vi "SCD - Generate FITS Timestamped File Paths.vi"(8 "error in":errorcluster, 11 "Base Path":path=path "G:/SCD Data/Level-0") -> (0 "error out":errorcluster, 3 "FITS File Path":path=path "G:/SCD Data/Level-0/20141031/20141031T094817.fits")   [LabVIEW 2014]
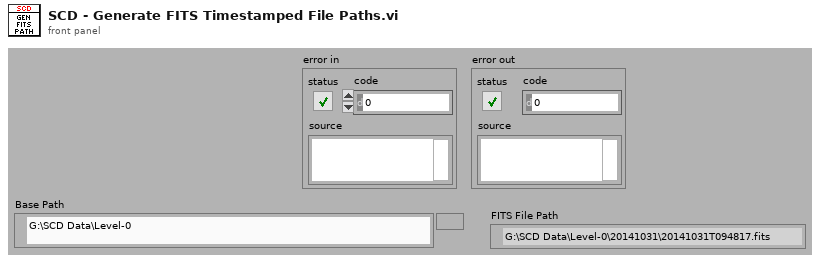
[diagram p1: front panel]
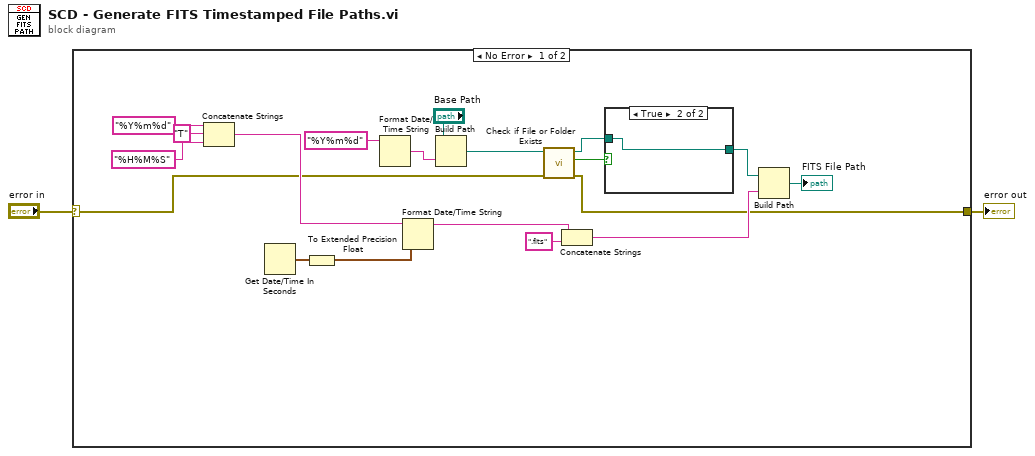
[diagram p0: block diagram]
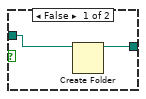
[diagram p2: hidden frame]
diagram:
  n1 = case shown="No Error" "error in" {
    selector: "error in" -> [w4 w24]
    tunnel: [w3 w24] -> w2
    frame No Error {
      n2 = Concatenate Strings("%Y%m%d" ("time format string (%c)"), "T" ("time format string (%c)"), "%H%M%S" ("time format string (%c)")) -> (w6:string)
      n3 = Get Date/Time In Seconds() -> (seconds since 1Jan1904=w10:timestamp)
      n4 = To Extended Precision Float(1:w10) -> ()  [unwired: 1 out]
      n5 = Format Date/Time String(time format string (%c)="%Y%m%d") -> (date/time string=w16:string)  [unwired: 2 out]
      n6 = Format Date/Time String(time format string (%c)=w6, seconds (now)=w10) -> (date/time string=w12:string)  [unwired: 1 in]
      n7 = Build Path(base path="Base Path", name or relative path=w16) -> (appended path=w19:path)
      n8 = call <vilib>:"Check if File or Folder Exists.vi"("error in (no error)"=w4, "path"=w19) -> ("error out"=w3:errorcluster, "file or folder exists?"=w13:bool, "dup path"=w18:path)  [unwired: 7 out]
      n9 = Concatenate Strings(w12, ".fits" ("string")) -> (w17:string)
      n10 = case shown="True" w13 {
        tunnel: [w22 w23] -> w11
        tunnel: w18 -> [w21 w23]
        frame False {
          n11 = Create Folder(path (use dialog)=w21) -> (created path=w22:path)  [unwired: 1 in, 3 out]
        }
        frame True {
        }
      }
      n12 = Build Path(base path=w11, name or relative path=w17) -> (appended path=→"FITS File Path":path)
    }
    frame Error {
    }
  }
  "error out" <- w2
